vi "Voltage against time to json 1 channel.vi"() -> ()   [LabVIEW 2015]
doc: "This example VI shows how to convert string data elements to numeric elements so it can be graphed and displayed on an XY Graph."
uses:
  <instrlib>/Keithley 27XX/Public/Data/Read Multiple Direct.vi
  <instrlib>/Keithley 27XX/Keithley 27XX.lvlib
panel:
  out "spreadsheet string":string
  in  "format string":string
  in  "delimiter (Tab)":string
  in  "file (use dialog)":path
  in  "Function (0: DC Voltage)":u16(ring) items=["DC Voltage", "AC Voltage", "DC Current", "AC Current", "Resistance", "Four-Wire Resistance", "Temperature (C)", "Frequency", "Period", "Continuity"]
  in  "Sample Count (10)":i32=10
  in  "Channel List (101:110)":string="101:110"
  out "XY Graph":T1(graph)
  in  "Serial Configuration":T2={"Baud Rate (9600)"=9600, "Flow Control (1: XON/XOFF)"=1, "Termination Char (0:CR)"=0} {"Termination Char (0:CR)" items=["CR", "LF", "CRLF (Do not use)", "LFCR (Do not use)"]; "Flow Control (1: XON/XOFF)" items=["None", "XON/XOFF", "RTS/CTS (2701 Only)", "XON/XOFF & RTS/CTS (2701 Only)"]; "Baud Rate (9600)" items=["300"=300, "600"=600, "1200"=1200, "2400"=2400, "4800"=4800, "9600"=9600, "19.2k"=19200, "38.4k (2701 Only)"=38400, "57.6k (2701 Only)"=57600, "115.2k (2701 Only)"=115200]}
  in  "Timeout (30000 milliseconds)":u32=30000
  in  "VISA resource name":refnum<visa-resource-name>
  # "© 2006 National Instruments Corporation.  ALL RIGHTS RESERVED."
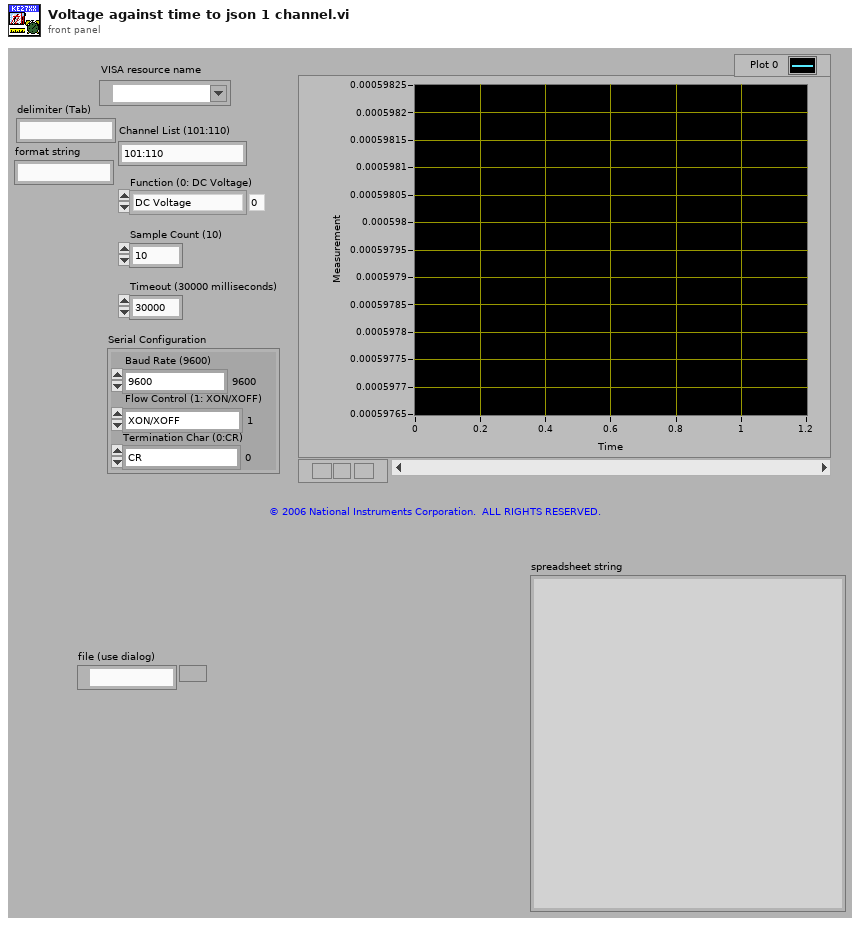
[diagram p1: front panel]
types:
  T1 = cluster{"Measurement Data":dbl[], "Converted Numeric Array":dbl[]}
  T2 = cluster{"Baud Rate (9600)":u32, "Flow Control (1: XON/XOFF)":u16, "Termination Char (0:CR)":u16}
  T3 = cluster{"Numeric Array":dbl[], "Measurement Data":dbl[]}
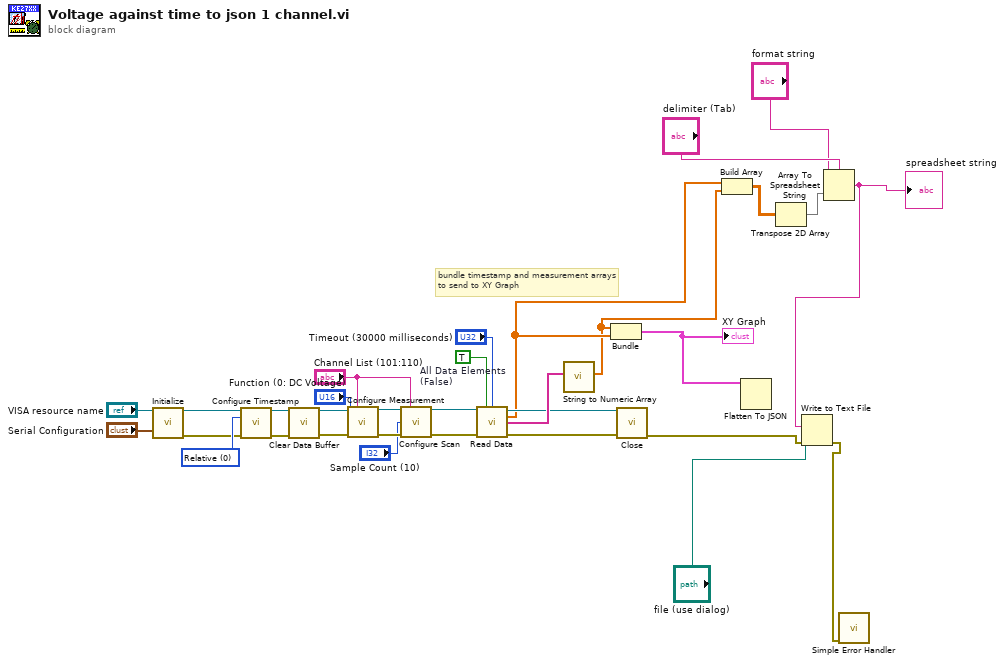
[diagram p0: block diagram]
diagram:
  w21 = u16 0 items=["Relative", "Real Time Clock"] ("Timestamp Type (0: Relative)")
  w31 = TRUE  # All Data Elements (False)
  # "bundle timestamp and measurement arrays to send to XY Graph"
  n1 = call <instrlib>:"Initialize.vi"("VISA resource name"="VISA resource name", "Serial Configuration"="Serial Configuration") -> ("VISA resource name out"=w18:refnum<visa-resource-name>, "error out"=w17:errorcluster)  [unwired: 12 in]
  n2 = call <instrlib>:"Configure Timestamp.vi"("VISA resource name"=w18, "Timestamp Type (0: Relative)"=w21, "error in (no error)"=w17) -> ("VISA resource name out"=w23:refnum<visa-resource-name>, "error out"=w22:errorcluster)  [unwired: 11 in]
  n3 = call <instrlib>:"Clear Data Buffer.vi"("VISA resource name"=w23, "error in (no error)"=w22) -> ("VISA resource name out"=w20:refnum<visa-resource-name>, "error out"=w24:errorcluster)  [unwired: 12 in]
  n4 = call <instrlib>:"Configure Measurement.vi"("VISA resource name"=w20, "Scan List (Empty)"="Channel List (101:110)", "Function (0: DC Voltage)"="Function (0: DC Voltage)", "error in (no error)"=w24) -> ("VISA resource name out"=w28:refnum<visa-resource-name>, "error out"=w26:errorcluster)  [unwired: 10 in]
  n5 = call <instrlib>:"Configure Scan.vi"("VISA resource name"=w28, "Channel List (101:110)"="Channel List (101:110)", "Sample Count (100)"="Sample Count (10)", "error in (no error)"=w26) -> ("VISA resource name out"=w16:refnum<visa-resource-name>, "error out"=w15:errorcluster)  [unwired: 10 in]
  n6 = call-poly <instrlib>:"Read Data.vi"("VISA resource name"=w16, "All Data Elements (False)"=w31, "Timeout (30000 milliseconds)"="Timeout (30000 milliseconds)", "error in (no error)"=w15) -> ("VISA resource name out"=w12:refnum<visa-resource-name>, "Measurement Data"=w7:dbl[], "Time Stamp"=w14:string[], "error out"=w13:errorcluster)  [unwired: 6 in, 2 out]
  n7 = call <instrlib>:"String to Numeric Array.vi"("String Array"=w14) -> ("Numeric Array"=w6:dbl[])  [unwired: 10 in]
  n8 = Bundle("Numeric Array"=w6, "Measurement Data"=w7) -> (w8:T3)  [unwired: 1 in]
  "XY Graph" <- w8
  n9 = call <instrlib>:"Close.vi"("VISA resource name"=w12, "error in (no error)"=w13) -> ("error out"=w10:errorcluster)  [unwired: 13 in]
  n10 = Build Array(w7, w6) -> (w2:dbl[][])
  n11 = Flatten To JSON(anything=w8) -> ()  [unwired: 2 in, 2 out]
  n12 = Transpose 2D Array(2D array=w2) -> (transposed array=w1:dbl[][])
  n13 = Array To Spreadsheet String(delimiter (Tab)="delimiter (Tab)", array=w1, 3:"format string") -> (spreadsheet string=w3:string)
  "spreadsheet string" <- w3
  n14 = Write to Text File(file (use dialog)="file (use dialog)", text=w3, error in=w10) -> (error out=w9:errorcluster)  [unwired: 1 in, 2 out]
  n15 = call <vilib>:"Simple Error Handler.vi"("error in (no error)"=w9) -> ()  [unwired: 4 in, 5 out]
